vi "PH_Cam_BaseClass.Draw Image.vi"(0 "i ref in":refnum<vi>, 5 "error in (no error)":errorcluster) -> (14 "i ref out":refnum<vi>, 19 "error out":errorcluster)   [LabVIEW 2014, in "PH_Cam_BaseClass.lvlib"]
uses:
  PH_Cam_BaseClass.lvlib
  <vilib>/vision/NI_Vision_Development_Module.lvlib
  CS_Core/CSSystem/CSSystemLib/CSSystemLib.lvlib
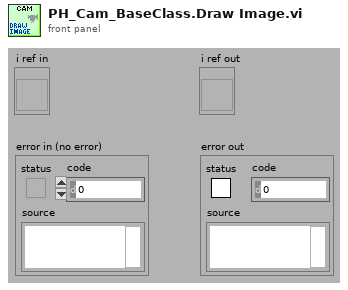
[diagram p1: front panel]
types:
  T1 = typedef "PH_Cam_BaseClass.lvlib/PH_Cam_BaseClass.i attribute.ctl" = cluster{"Gui Refs":T2, "Cam":cluster{"Source Notifier":refnum<notifier>, "Error":errorcluster, "Camera ID":string}, "Images":cluster{"Cam":T3, "Operation":T3, "PSDB":T3}, "Window Image":cluster{"Indicate Image":bool, "Window No.":i32, "Scale Facor":dbl, "Center Cross":bool, "Subtract Backgr":bool, "CoG":bool, "Color Palette":cluster{"Red":u8, "Green":u8, "Blue":u8}[], "Image On":bool}, "Default Prdc Int":i32, "Performance":cluster{"on":bool, "Timestamp Last Frame":i32}, "Histogram":cluster{"on":bool, "Mapping":bool}, "Save Image":cluster{"Save":bool, "File refnum":refnum<file>}, "Setting Service ID":i32, "Screen":cluster{"x-resolution":i16, "y-resolution":i16}, "On":bool, "Constructor finished":bool, "configured":bool}
  T2 = typedef "PH_Cam_BaseClass.lvlib/PH_Cam_BaseClass.GUI Refs.ctl" = cluster{"Frame Rate":refnum<vi>, "Get Frame Rate":refnum<vi>, "Show Image":refnum<vi>, "Get Histogram":refnum<vi>, "Mapping":refnum<vi>, "Histogram":refnum<vi>, "Center Cross":refnum<vi>, "Center of Gravity":refnum<vi>, "Scale Factor [%]":refnum<vi>, "Save Image":refnum<vi>, "Palette":refnum<vi>, "Subtract Background":refnum<vi>, "Cam Error":refnum<vi>, "On":refnum<vi>, "Cam List":refnum<vi>}
  T3 = typedef "IMAQ Image.ctl" = refnum<image>
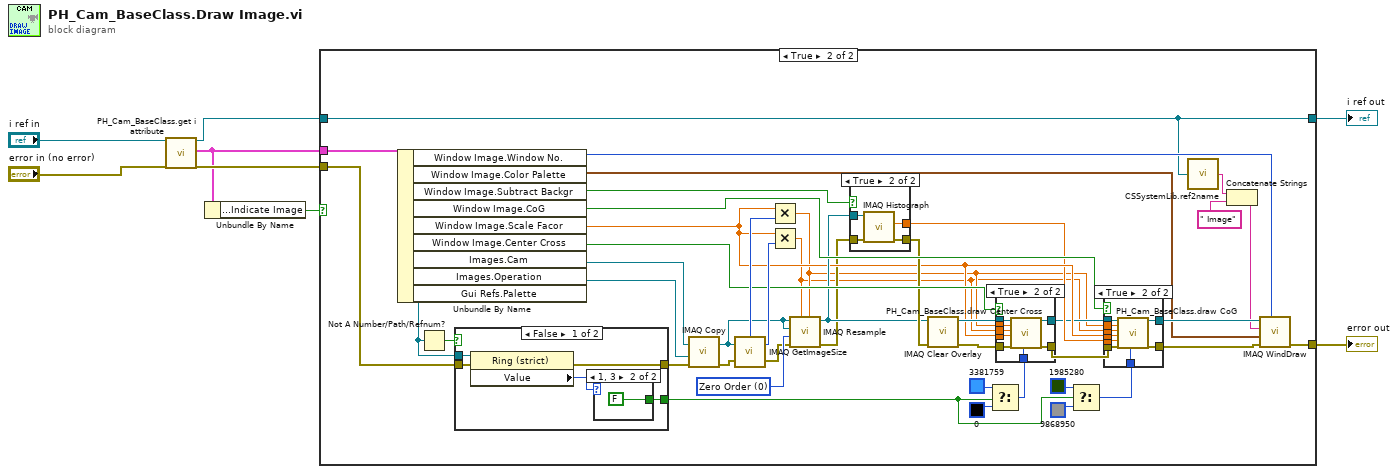
[diagram p0: block diagram]
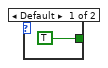
[diagram p3: hidden frame]
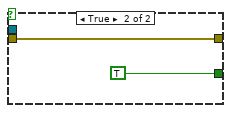
[diagram p4: hidden frame]
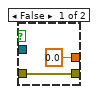
[diagram p7: hidden frame]
diagram:
  n1 = call "PH_Cam_BaseClass.get i attribute.vi"("i ref in"="i ref in", "error in (no error)"="error in (no error)") -> ("i ref out"=w2:refnum<vi>, "i attribute"=w5:T1, "error out"=w8:errorcluster)  [unwired: 15 in]
  n2 = Unbundle By Name(w5) -> ("Window Image.Indicate Image"=w3:bool)
  n3 = case shown="True" w3 {
    tunnel: w8 -> [w9 w49]
    tunnel: [w9 w25] -> w7
    tunnel: w5 -> [_ w21]
    tunnel: w2 -> [w10 w13]
    tunnel: [w10 w13] -> w1
    frame False {
    }
    frame True {
      w23 = u32 0 items=["Zero Order", "Bi-Linear", "Quadratic", "Cubic Spline"] ("Interpolation Type")
      n4 = Unbundle By Name(w21) -> ("Window Image.Window No."=w17:i32, "Window Image.Color Palette"=w29:cluster{"Red":u8, "Green":u8, "Blue":u8}[], "Window Image.Subtract Backgr"=w26:bool, "Window Image.CoG"=w48:bool, "Window Image.Scale Facor"=w33:dbl, "Window Image.Center Cross"=w42:bool, "Images.Cam"=w12:T3, "Images.Operation"=w11:T3, "Gui Refs.Palette"=w51:refnum<vi>)
      n5 = Not A Number/Path/Refnum?(number/path/refnum=w51) -> (NaN/Path/Refnum?=w52:bool)
      n6 = case shown="False" w52 {
        tunnel: w49 -> [w58 w61]
        tunnel: [w57 w61] -> w50
        tunnel: w51 -> [w56 _]
        tunnel: [w54 TRUE] -> w53
        frame False {
          n7 = property class="Ring (strict)"(reference=w56, error in=w58) -> (error out=w57:errorcluster, "Value"=w55:i32)  [unwired: 1 out]
          n8 = case shown="1, 3" w55 {
            tunnel: [TRUE FALSE] -> w54
            frame Default {
            }
            frame 1, 3 {
            }
          }
        }
        frame True {
        }
      }
      n9 = call "IMAQ Copy"("error in (no error)"=w50, "Image Dst"=w11, "Image Src"=w12) -> ("error out"=w27:errorcluster, "Image Dst Out"=w28:T3)  [unwired: 3 in]
      n10 = call "IMAQ GetImageSize"("Image"=w28, "error in (no error)"=w27) -> ("Y Resolution"=w46:i32, "X Resolution"=w47:i32, "error out"=w22:errorcluster)  [unwired: 2 in]
      n11 = Multiply(x=w33, y=w47) -> (x*y=w16:dbl)
      n12 = Multiply(x=w33, y=w46) -> (x*y=w15:dbl)
      n13 = call "IMAQ Resample"("X Resolution"=w16, "Y Resolution"=w15, "error in (no error)"=w22, "Interpolation Type"=w23, "Image Dst"=w28, "Image Src"=w28) -> ("error out"=w24:errorcluster, "Image Dst Out"=w35:T3)  [unwired: 4 in]
      n14 = case shown="True" w26 {
        tunnel: w35 -> [_ w89]
        tunnel: w24 -> [w84 w88]
        tunnel: [w84 w87] -> w38
        tunnel: [sgl 0.0 ("Mean Value") w86] -> w32
        frame False {
        }
        frame True {
          n15 = call "IMAQ Histograph"("error in (no error)"=w88, "Image"=w89) -> ("error out"=w87:errorcluster, "Mean Value"=w86:sgl)  [unwired: 6 in, 2 out]
        }
      }
      n16 = call "IMAQ Clear Overlay"("error in (no error)"=w38, "Image"=w35) -> ("error out"=w37:errorcluster, "Image Out"=w36:T3)  [unwired: 8 in]
      n17 = Select(t=u32 3381759 ("Color"), s=w53, f=u32 0 ("Color")) -> (s? t:f=w41:u32)
      n18 = case shown="True" w42 {
        tunnel: [w74 w83] -> w30
        tunnel: [w75 w82] -> w31
        tunnel: w33 -> [_ w81]
        tunnel: w36 -> [w75 w80]
        tunnel: w37 -> [w74 w79]
        tunnel: w41 -> [_ w78]
        tunnel: w16 -> [_ w77]
        tunnel: w15 -> [_ w76]
        frame False {
        }
        frame True {
          n19 = call "PH_Cam_BaseClass.draw Center Cross.vi"("Image In"=w80, "X Resolution"=w77, "Y Resolution"=w76, "Scale Factor"=w81, "error in (no error)"=w79, "Color"=w78) -> ("Image Out"=w82:T3, "error out"=w83:errorcluster)  [unwired: 12 in]
        }
      }
      n20 = Select(t=u32 1985280 ("Color"), s=w53, f=u32 9868950 ("Color")) -> (s? t:f=w45:u32)
      n21 = case shown="True" w48 {
        tunnel: w30 -> [w63 w73]
        tunnel: w31 -> [w64 w72]
        tunnel: w32 -> [_ w71]
        tunnel: w33 -> [_ w70]
        tunnel: [w64 w69] -> w34
        tunnel: [w63 w68] -> w14
        tunnel: w45 -> [_ w67]
        tunnel: w15 -> [_ w66]
        tunnel: w16 -> [_ w65]
        frame False {
        }
        frame True {
          n22 = call "PH_Cam_BaseClass.draw CoG.vi"("Image In"=w72, "X Resolution"=w65, "Y Resolution"=w66, "Scale Factor"=w70, "Background Offset"=w71, "error in (no error)"=w73, "Color"=w67) -> ("Image Out"=w69:T3, "error out"=w68:errorcluster)  [unwired: 11 in]
        }
      }
      n23 = call "CSSystemLib.ref2name.vi"("obj refnum"=w13) -> ("name"=w20:string)
      n24 = Concatenate Strings(w20, " Image" ("string")) -> (w18:string)
      n25 = call "IMAQ WindDraw"("Window Number (0...15)"=w17, "error in (no error)"=w14, "Color Palette"=w29, "Title"=w18, "Image"=w34) -> ("error out"=w25:errorcluster)  [unwired: 5 in, 1 out]
    }
  }
  "error out" <- w7
  "i ref out" <- w1
